vi "Write SV.vi"(8 "error in (no error)":errorcluster, 10 "Data":dbl[](array[numeric]), 11 "Write Refs by Type":cluster{"DBL Write":refnum<k21>[]}) -> (0 "error out":errorcluster)   [LabVIEW 2020, in "Shared Variable Interface.lvlib"]
uses:
  Shared Variable Interface.lvlib
  DataTypes/DBL.lvlib
  <vilib>/Utility/Variable/NI_VariableUtilities.lvlib
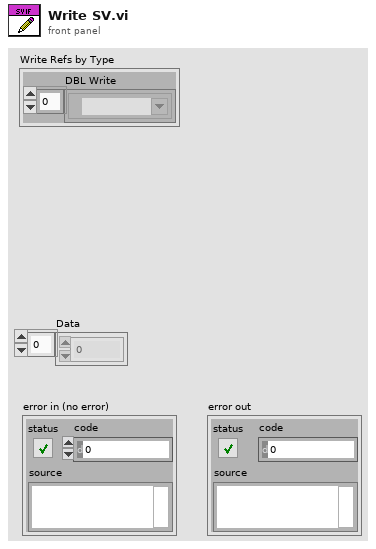
[diagram p1: front panel]
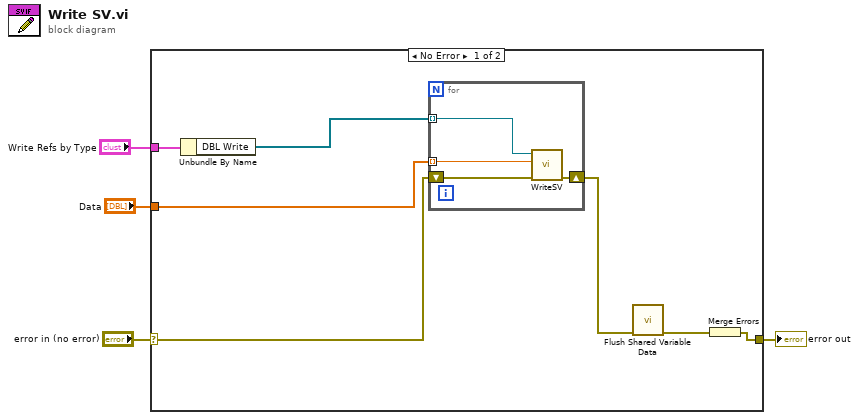
[diagram p0: block diagram]
diagram:
  n1 = case shown="No Error" "error in (no error)" {
    selector: "error in (no error)" -> [w9 w16]
    tunnel: [w11 w16] -> w4
    tunnel: "Data" -> [w7 _]
    tunnel: "Write Refs by Type" -> [w8 _]
    frame No Error {
      n2 = Unbundle By Name(w8) -> ("DBL Write"=w10:refnum<k21>[])
      n3 = for {
        tunnel: w10 -> [w13] mode=indexing
        shift-right: [w14] -> w6
        shift-left: w9 -> [w15]
        tunnel: w7 -> [w12] mode=indexing
        n4 = call "WriteSV.vi"("error in (no error)"=w15, "DBL Data"=w12, "shared variable refnum in"=w13) -> ("error out"=w14:errorcluster)  [unwired: 8 in]
      }
      n5 = call <vilib>:"Flush Shared Variable Data.vi"("error in (no error)"=w6) -> ("error out"=w5:errorcluster)  [unwired: 10 in]
      n6 = Merge Errors(w5) -> (w11:errorcluster)
    }
    frame Error {
    }
  }
  "error out" <- w4
